vi "Find Center Angle in Degrees.vi"(7 "output range (-180 to 180)":T1=enum."-180 to 180", 9 "right angle (deg)":dbl, 11 "left angle (deg)":dbl) -> (2 "center angle (deg)":dbl)   [LabVIEW 2017, in "NI_Robotics Utilities.lvlib"]
doc: "This VI is deprecated. Use <vi.lib>\\Analysis\\coordinate.llb\\Find Center Angle.vi instead."
uses:
  <vilib>/robotics/Utilities/NI_Robotics Utilities.lvlib
  <vilib>/robotics/Utilities/Angle Range_Degrees.ctl
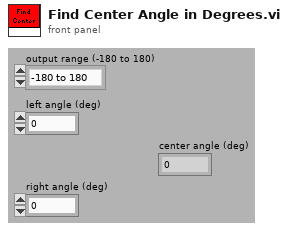
[diagram p1: front panel]
types:
  T1 = typedef "NI_Robotics Utilities.lvlib/Angle Range_Degrees.ctl" = enum16{"none", "-180 to 180", "0 to 360"}
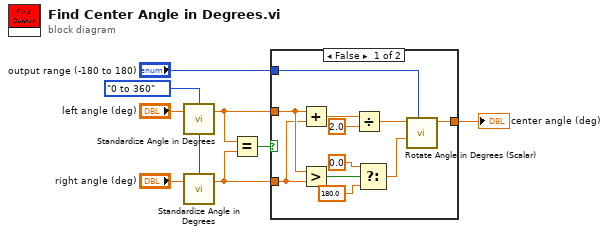
[diagram p0: block diagram]
diagram:
  w2 = Angle_Range_Degrees."0 to 360" ("range (-180 to 180)")
  n1 = call <vilib>:"Standardize Angle in Degrees.vi"("angle in (deg)"="left angle (deg)", "range (-180 to 180)"=w2) -> ("angle out (deg)"=w6:dbl)  [unwired: 3 in]
  n2 = call <vilib>:"Standardize Angle in Degrees.vi"("angle in (deg)"="right angle (deg)", "range (-180 to 180)"=w2) -> ("angle out (deg)"=w5:dbl)  [unwired: 3 in]
  n3 = Equal?(x=w6, y=w5) -> (x = y?=w4:bool)
  n4 = case shown="False" w4 {
    tunnel: [w10 w20] -> w1
    tunnel: w5 -> [w17 _]
    tunnel: w6 -> [w18 w20]
    tunnel: "output range (-180 to 180)" -> [w11 _]
    frame False {
      n5 = Add(x=w18, y=w17) -> (x+y=w19:dbl)
      n6 = Greater?(x=w18, y=w17) -> (0:w15:bool)
      n7 = Divide(x=w19, y=2.0) -> (x/y=w13:dbl)
      n8 = Select(t=0.0, s=w15, f=180.0) -> (s? t:f=w12:dbl)
      n9 = call <vilib>:"Rotate Angle in Degrees (Scalar).vi"("output range (-180 to 180)"=w11, "ccw rotation (deg)"=w12, "angle in (deg)"=w13) -> ("angle out (deg)"=w10:dbl)  [unwired: 8 in]
    }
    frame True {
    }
  }
  "center angle (deg)" <- w1
